vi "利用余弦定理求三角形内角.vi"(0 "c":dbl=5.0, 1 "b":dbl=4.0, 2 "a":dbl=3.0) -> ()   [LabVIEW 2012, in "几何工具.lvlib"]
doc: "功能：\n\n利用余弦定理求三角形内角。\n\n公式：\n\n三角形三边分别为a b c，函数返回c边所对的内角，单位为度。\n\ncos(c)=(a^2+b^2-c^2)/(2*a*b)"
panel:
  out "CAngle":dbl=5.0
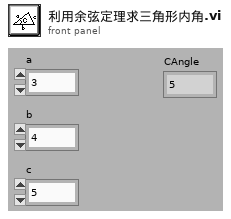
[diagram p1: front panel]
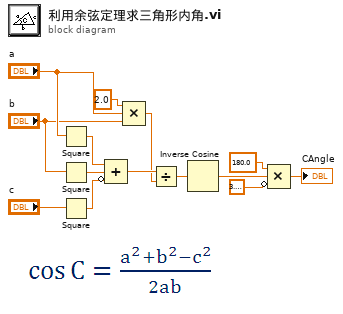
[diagram p0: block diagram]
diagram:
  n1 = Square(x="a") -> (x^2=w10:dbl)
  n2 = Square(x="b") -> (x^2=w9:dbl)
  n3 = Square(x="c") -> (x^2=w2:dbl)
  n4 = Compound Arithmetic op=ADD(w10, w9, invert w2) -> (w8:dbl)
  n5 = Compound Arithmetic op=MULTIPLY(2.0 ("值"), "a", "b") -> (w1:dbl)
  n6 = Divide(x=w8, y=w1) -> (x/y=w7:dbl)
  n7 = Inverse Cosine(1:w7) -> (0:w5:dbl)
  n8 = Compound Arithmetic op=MULTIPLY(180.0 ("值"), w5, invert 3.141592653589793) -> (→"CAngle":dbl)
